vi "tcpServerCallBack.vi"(8 "error in (no error)":errorcluster, 11 "TcpServerTel in":refnum<class "TcpServerTel.lvclass">) -> (0 "error out":errorcluster, 3 "TcpServerTel out":refnum<class "TcpServerTel.lvclass">)   [LabVIEW 2018, in "TcpServerTel.lvclass"]
doc: "Receive the incoming json command from TCP Client and process it, and send the results in a queue to the LabVIEW Component."
uses:
  TcpServerTel.lvclass
  home/pcortes/github/ts_labview_tcp_json/src/TcpServerBase/TcpServerBase.lvclass
  TcpServerBase/TcpServerBase.lvclass/TcpServerBase.ctl
  TcpServerBase/TcpServerBase.lvclass
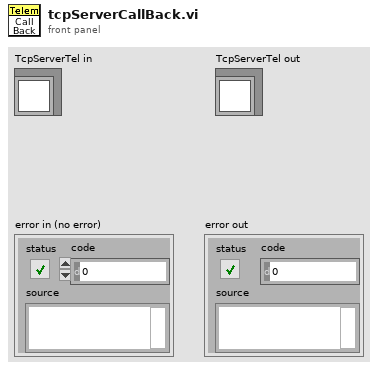
[diagram p1: front panel]
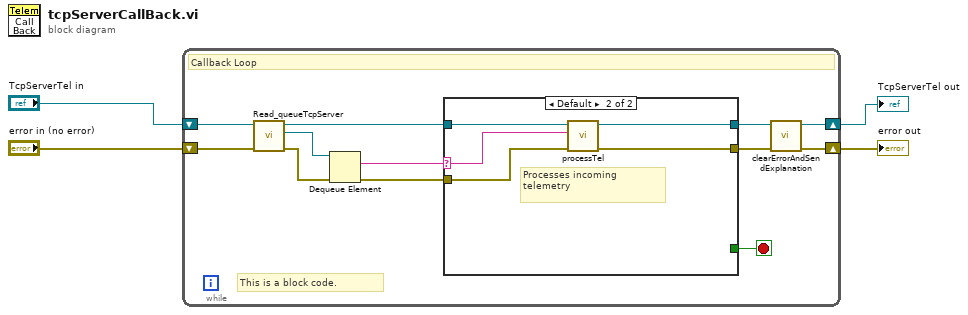
[diagram p0: block diagram]
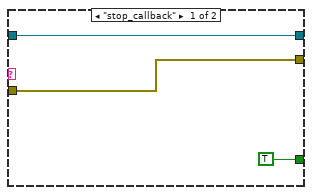
[diagram p2: hidden frame]
diagram:
  n1 = while {
    shift-right: [w8] -> w4
    shift-left: "error in (no error)" -> [w14]
    shift-right: [w6] -> w1
    shift-left: "TcpServerTel in" -> [w15]
    stop <- w5 stop-if-true
    # "This is a block code."
    # "Callback Loop"
    n2 = call "Read_queueTcpServer.vi"("error in (no error)"=w14, "TcpServerBase in"=w15) -> ("error out"=w10:errorcluster, "queueTcpServer"=w16:refnum<queue>, "TcpServerBase out"=w12:refnum<class "TcpServerTel.lvclass">)  [unwired: 7 in]
    n3 = Dequeue Element(queue=w16, error in (no error)=w10) -> (element=w11:string, error out=w9:errorcluster)  [unwired: 1 in, 2 out]
    n4 = case shown="Default" w11 {
      selector: w11 -> [_ w20]
      tunnel: w12 -> [w18 w24]
      tunnel: [TRUE _] -> w5
      tunnel: [w17 w23] -> w13
      tunnel: [w18 w22] -> w7
      tunnel: w9 -> [w17 w21]
      frame "stop_callback" {
      }
      frame Default {
        # "Processes incoming\ntelemetry"
        n5 = call "processTel.vi"("error in (no error)"=w21, "packet"=w20, "TcpServerTel in"=w24) -> ("error out"=w23:errorcluster, "TcpServerTel out"=w22:refnum<class "TcpServerTel.lvclass">)  [unwired: 7 in]
      }
    }
    n6 = call "clearErrorAndSendExplanation.vi"("error in (no error)"=w13, "TcpServerBase in"=w7) -> ("error out"=w8:errorcluster, "TcpServerBase out"=w6:refnum<class "TcpServerTel.lvclass">)  [unwired: 8 in]
  }
  "error out" <- w4
  "TcpServerTel out" <- w1
